vi "isPrivate.vi"(8 "error in (no error)":errorcluster, 11 "Element in":refnum<class "Element.lvclass">) -> (0 "error out":errorcluster, 2 "isPrivate":bool, 3 "Element out":refnum<class "Element.lvclass">)   [LabVIEW 2016, in "Element.lvclass"]
uses:
  Element.lvclass
  Element.lvclass/Element.ctl
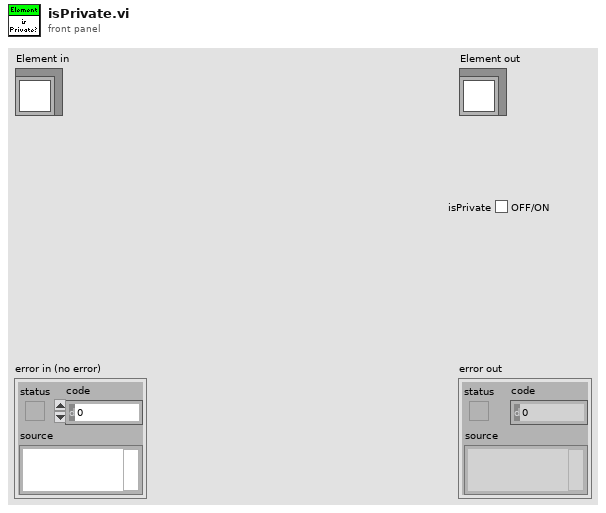
[diagram p1: front panel]
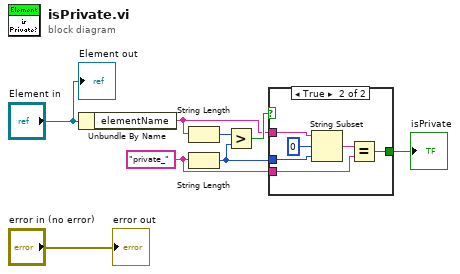
[diagram p0: block diagram]
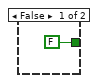
[diagram p2: hidden frame]
diagram:
  w4 = "private_"
  n1 = Unbundle By Name("Element in") -> ("elementName"=w5:string)
  n2 = String Length(string=w5) -> (length=w8:i32)
  n3 = String Length(string=w4) -> (length=w6:i32)
  n4 = Greater?(x=w8, y=w6) -> (0:w7:bool)
  n5 = case shown="True" w7 {
    tunnel: w6 -> [_ w14]
    tunnel: w5 -> [_ w13]
    tunnel: w4 -> [_ w11]
    tunnel: [FALSE w10] -> w3
    frame False {
    }
    frame True {
      n6 = String Subset(string=w13, offset (0)=0, length (rest)=w14) -> (substring=w12:string)
      n7 = Equal?(x=w12, y=w11) -> (x = y?=w10:bool)
    }
  }
  "isPrivate" <- w3
  "error out" <- "error in (no error)"
  "Element out" <- "Element in"
